vi "Dashboard to Center.vi"(8 "error in (no error)":errorcluster, 11 "Control Ref":refnum<vi>) -> (0 "error out":errorcluster)   [LabVIEW 2020, in "CSM-TagDashboard.lvlib"]
uses:
  CSM-TagDashboard.lvlib
  <vilib>/Utility/miscctls.llb/LVRectTypeDef.ctl
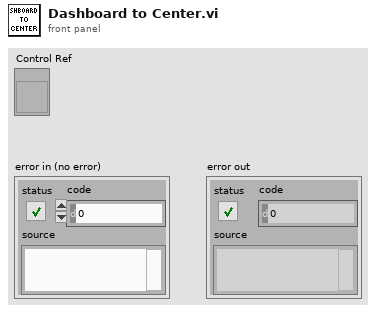
[diagram p1: front panel]
types:
  T1 = typedef "LVRectTypeDef.ctl" = cluster{"Left":i16, "Top":i16, "Right":i16, "Bottom":i16}
  T2 = typedef "LVBoundsTypeDef.ctl" = cluster{"Width":u32, "Height":u32}
  T3 = cluster{"left":i16, "top":i16, "right":i16, "bottom":i16}
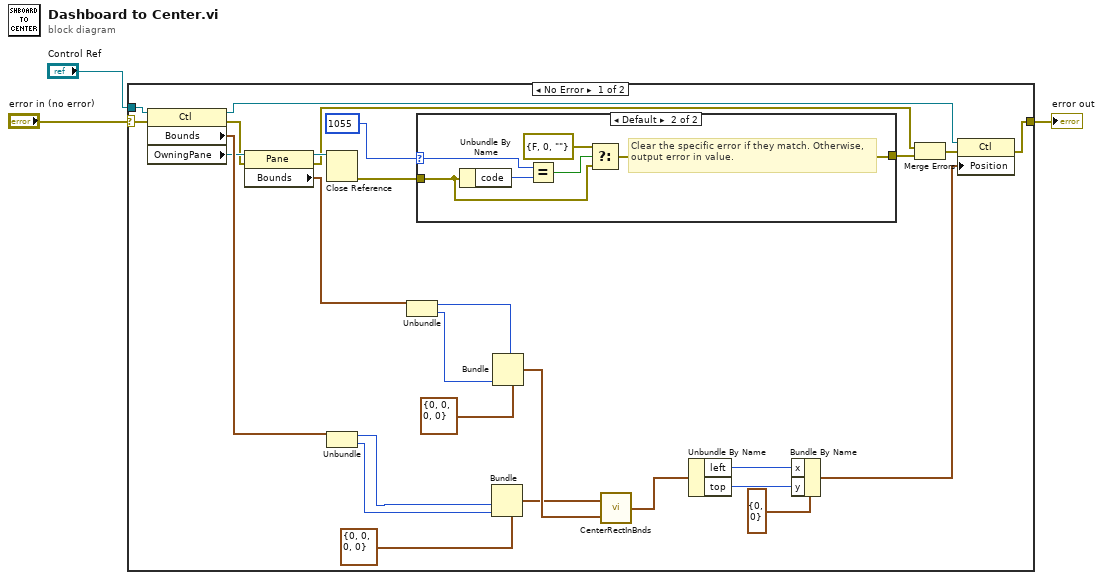
[diagram p0: block diagram]
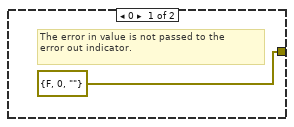
[diagram p2: hidden frame]
diagram:
  n1 = case shown="No Error" "error in (no error)" {
    selector: "error in (no error)" -> [w27 w38]
    tunnel: "Control Ref" -> [w30 _]
    tunnel: [w25 w38] -> w1
    frame No Error {
      n2 = property class="Ctl"(reference=w30, error in=w27) -> (reference out=w29:refnum<vi>, error out=w20:errorcluster, "Bounds"=w28:T2, "OwningPane"=w24:refnum<vi>)
      n3 = property class="Pane"(reference=w24, error in=w20) -> (reference out=w19:refnum<vi>, error out=w18:errorcluster, "Bounds"=w23:T2)
      n4 = Close Reference(reference=w19) -> (error out=w14:errorcluster)  [unwired: 1 in]
      n5 = Unbundle(w28) -> ("Width"=w8:u32, "Height"=w7:u32)
      n6 = Unbundle(w23) -> ("Width"=w5:u32, "Height"=w4:u32)
      n7 = case shown="Default" 1055 ("specific error code to clear (0: all)") {
        selector: 1055 ("specific error code to clear (0: all)") -> [_ w36]
        tunnel: w14 -> [_ w35]
        tunnel: [errorcluster {"status"=FALSE, "code"=0, "source"=""} ("error constant") w32] -> w15
        frame 0 {
          # "The error in value is not passed to the\nerror out indicator."
        }
        frame Default {
          # "Clear the specific error if they match. Otherwise, output error in value."
          n8 = Unbundle By Name(w35) -> ("code"=w37:i32)
          n9 = Equal?(x=w36, y=w37) -> (x = y?=w33:bool)
          n10 = Select(t=errorcluster {"status"=FALSE, "code"=0, "source"=""} ("error constant"), s=w33, f=w35) -> (s? t:f=w32:errorcluster)
        }
      }
      n11 = Bundle(cluster=T1 {"Left"=0, "Top"=0, "Right"=0, "Bottom"=0} ("Windows Bounds"), "Right"=w8, "Bottom"=w7) -> (w21:T1)  [unwired: 2 in]
      n12 = Bundle(cluster=T1 {"Left"=0, "Top"=0, "Right"=0, "Bottom"=0} ("Windows Bounds"), "Right"=w5, "Bottom"=w4) -> (w22:T1)  [unwired: 2 in]
      n13 = call <vilib>:"CenterRectInBnds.vi"("bounds"=w22, "rect"=w21) -> ("centered rect"=w13:T3)
      n14 = Unbundle By Name(w13) -> ("left"=w11:i16, "top"=w12:i16)
      n15 = Bundle By Name(cluster=cluster{"x":i32, "y":i32} {"x"=0, "y"=0} ("Point"), "x"=w11, "y"=w12) -> (w26:cluster{"x":i32, "y":i32})
      n16 = Merge Errors(w18, w15) -> (w17:errorcluster)
      n17 = property class="Ctl"(reference=w29, error in=w17, "Position"=w26) -> (error out=w25:errorcluster)  [unwired: 1 out]
    }
    frame Error {
    }
  }
  "error out" <- w1
